vi "GetData.vi"(9 "VarTree_in":T1 {"Rawdata" format="0x%08x"}, 10 "InputsRate":i32=380, 11 "Conn":T4) -> (0 "error out":errorcluster, 1 "VarTree_out":T1 {"Rawdata" format="0x%08x"}, 2 "DataStats":T5, 3 "Conn_Problem?":bool)   [LabVIEW 2014]
uses:
  type_def/DataCluster.ctl
  ConsCluster.ctl
  _init_vartree/typedefs/ExVarTreeArray.ctl
  _init_vartree/typedefs/ExVarTree.ctl
  _init_vartree/typedefs/val_type_t.ctl
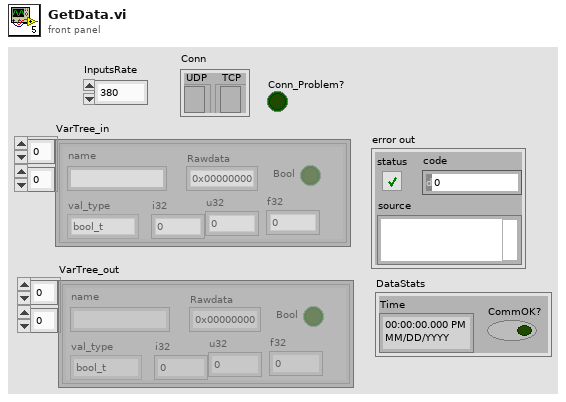
[diagram p1: front panel]
types:
  T1 = typedef "ExVarTreeArray.ctl" = T2[][]
  T2 = typedef "ExVarTree.ctl" = cluster{"name":string, "val_type":T3, "Rawdata":u32, "i32":i32, "u32":u32, "f32":sgl, "Bool":bool}
  T3 = typedef "val_type_t.ctl" = enum16{"bool_t", "i32_t", "u32_t", "f32_t"}
  T4 = typedef "ConsCluster.ctl" = cluster{"UDP":refnum<k16>, "TCP":refnum<k5>}
  T5 = typedef "DataCluster.ctl" = cluster{"Time":timestamp, "CommOK?":bool}
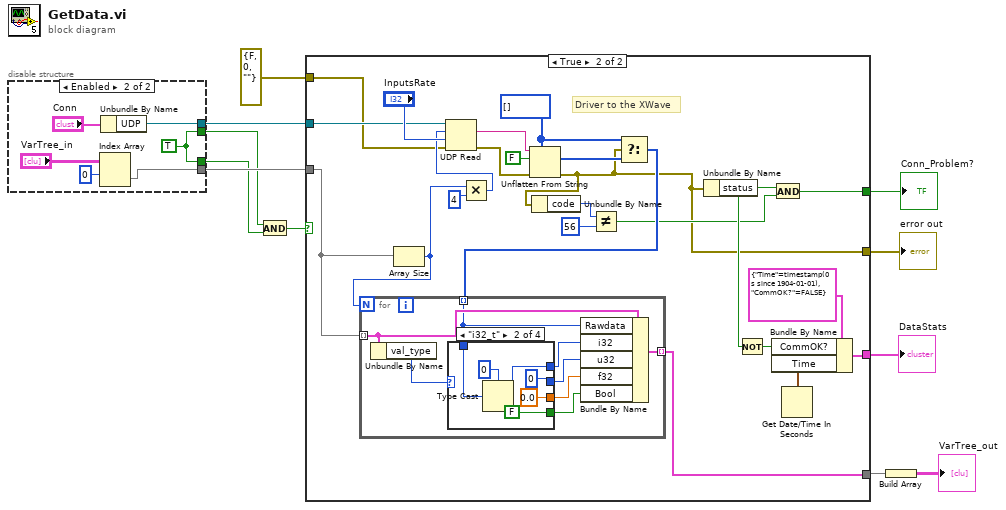
[diagram p0: block diagram]
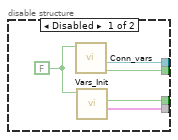
[diagram p2: hidden frame]
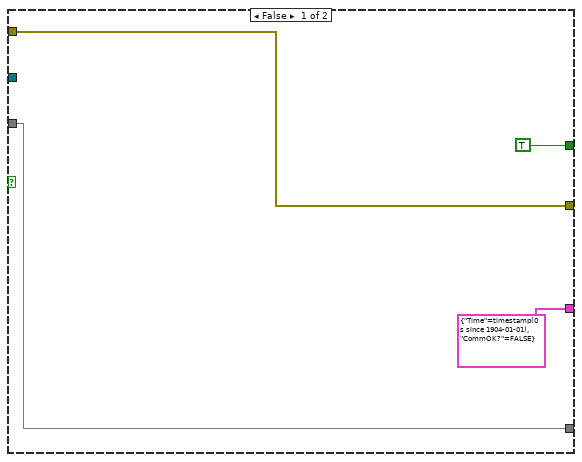
[diagram p3: hidden frame]
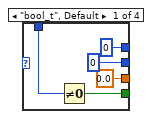
[diagram p4: hidden frame]
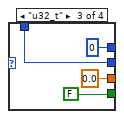
[diagram p5: hidden frame]
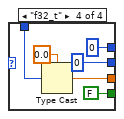
[diagram p6: hidden frame]
diagram:
  n1 = disable-structure shown="Enabled" {
    disable-tunnel: [w16 w17] -> w9
    disable-tunnel: [w15 w21] -> w8
    disable-tunnel: [w14 w20] -> w6
    disable-tunnel: [w13 w20] -> w5
    frame Disabled {
      w12 = FALSE ("WriteVars?")
      n2 = call "Conn_vars.vi"("WriteVars?"=w12) -> ("Connected_Out"=w14:bool, "UDPConnOut"=w15:refnum<k16>)  [unwired: 8 in, 1 out]
      n3 = call "Vars_Init.vi"("WriteVars?"=w12) -> ("Data Cluster Out"=w16:T5, "Init? Out"=w13:bool)  [unwired: 9 in]
    }
    frame Enabled {
      w20 = TRUE
      n4 = Index Array(array="VarTree_in", index (row)=0) -> (element=w17:T2[])  [unwired: 1 in]
      n5 = Unbundle By Name("Conn") -> ("UDP"=w21:refnum<k16>)
    }
  }
  n6 = And(x=w6, y=w5) -> (x .and. y?=w7:bool)
  n7 = case shown="True" w7 {
    tunnel: [T5 {"Time"=timestamp(0 s since 1904-01-01), "CommOK?"=FALSE} ("DataStats") w30] -> w3
    tunnel: [w25 w35] -> w11
    tunnel: [TRUE w34] -> w10
    tunnel: w9 -> [w23 w29]
    tunnel: w8 -> [_ w33]
    tunnel: errorcluster {"status"=FALSE, "code"=0, "source"=""} ("error in (no error)") -> [w25 w32]
    tunnel: [w23 w27] -> w2
    frame False {
    }
    frame True {
      w50 = u32[] [] ("sysvars")
      # "Driver to the XWave"
      n8 = Array Size(array=w29) -> (size(s)=w28:i32)
      n9 = Multiply(x=w28, y=4) -> (x*y=w42:i32)
      n10 = UDP Read(connection ID=w33, max size (548)=w42, timeout ms (25000)="InputsRate", 8:w32) -> (data out=w36:string, error out=w41:errorcluster)  [unwired: 3 out]
      n11 = Unflatten From String(type=w50, binary string=w36, data includes array or string size? (T)=FALSE, error in (no error)=w41) -> (value=w39:u32[], error out=w35:errorcluster)  [unwired: 1 in, 1 out]
      n12 = Unbundle By Name(w35) -> ("code"=w37:i32)
      n13 = Not Equal?(x=w37, y=56) -> (x != y?=w44:bool)
      n14 = Select(t=w50, s=w35, f=w39) -> (s? t:f=w45:u32[])
      n15 = for {
        N: w28 -> [_]
        tunnel: w45 -> [w55] mode=indexing
        tunnel: w29 -> [w57] mode=indexing
        tunnel: [w58] -> w27 mode=indexing
        n16 = Unbundle By Name(w57) -> ("val_type"=w56:T3)
        n17 = case shown="\"i32_t\"" w56 {
          tunnel: w55 -> [w63 w69 w73 w77]
          tunnel: [0 w67 0 0] -> w54
          tunnel: [u32 0 u32 0 w73 u32 0] -> w53
          tunnel: [sgl 0.0 sgl 0.0 sgl 0.0 w78] -> w52
          tunnel: [w62 FALSE FALSE FALSE] -> w51
          frame "bool_t", Default {
            n18 = Not Equal To 0?(x=w63) -> (x != 0?=w62:bool)
          }
          frame "i32_t" {
            n19 = Type Cast(type=0, x=w69) -> (*(type *) &x=w67:i32)
          }
          frame "u32_t" {
          }
          frame "f32_t" {
            n20 = Type Cast(type=sgl 0.0, x=w77) -> (*(type *) &x=w78:sgl)
          }
        }
        n21 = Bundle By Name(cluster=w57, "Rawdata"=w55, "i32"=w54, "u32"=w53, "f32"=w52, "Bool"=w51) -> (w58:T2)
      }
      n22 = Unbundle By Name(w35) -> ("status"=w48:bool)
      n23 = Not(x=w48) -> (.not. x?=w49:bool)
      n24 = And(x=w48, y=w44) -> (x .and. y?=w34:bool)
      n25 = Get Date/Time In Seconds() -> (seconds since 1Jan1904=w46:timestamp)
      n26 = Bundle By Name(cluster=T5 {"Time"=timestamp(0 s since 1904-01-01), "CommOK?"=FALSE} ("DataStats"), "CommOK?"=w49, "Time"=w46) -> (w30:T5)
    }
  }
  "DataStats" <- w3
  "error out" <- w11
  "Conn_Problem?" <- w10
  n27 = Build Array(w2) -> (→"VarTree_out":T2[][])
